vi "SDI_Single-Axis_Test.vi"() -> ()   [LabVIEW 2014]
uses:
  <vilib>/Motion/plugins/PluginFramework/nismSDIFramework.SetFrameworkMode.single.vi
  <vilib>/Motion/Express/_s/nimc.ex.clearFaults.clearFaults.axis.vi
  <vilib>/Motion/Express/_s/nimc.ex.power.power.axis.vi
  <vilib>/Motion/BlockNode/FB.NIMotion.xnode
  <vilib>/Motion/plugins/Delta ASDA SDI Plug-in/Template SoftMotion Drive Interface Plug-in Class.lvclass
panel:
  out "error out":errorcluster
  in  "stop":bool
  in  "Axis":refnum<k21>="Axis 1"
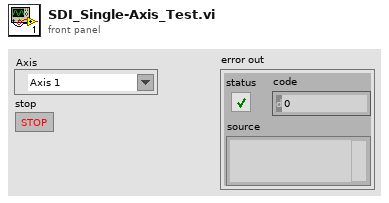
[diagram p1: front panel]
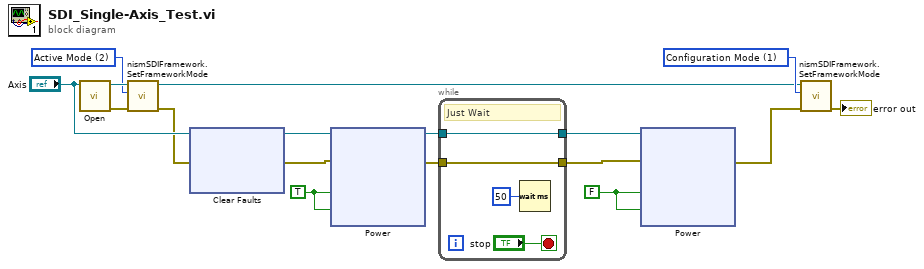
[diagram p0: block diagram]
diagram:
  w8 = 1 items=["Configuration Mode"=1, "Active Mode"=2] ("mode (Active Mode)")
  w11 = FALSE ("enable axis")
  w14 = TRUE ("enable axis")
  w16 = 2 items=["Configuration Mode"=1, "Active Mode"=2] ("mode (Active Mode)")
  n1 = call <vilib>:"Open.vi"("Axis"="Axis") -> ("error out"=w15:errorcluster, "Base Axis Out"=w17:refnum<class "nismPluginAxisBaseClass.lvclass">)  [unwired: 9 in]
  n2 = call-poly <vilib>:"nismSDIFramework.SetFrameworkMode.vi"("error in (no error)"=w15, "mode (Active Mode)"=w16, "Base Axis In"=w17) -> ("error out"=w3:errorcluster, "Base Axis Out"=w7:refnum<class "nismPluginAxisBaseClass.lvclass">)  [unwired: 7 in]
  n3 = xnode ("Clear Faults")("resource"="Axis", "error in"=w3) -> ("resource out"=w2:refnum<k21>, "error out"=w1:errorcluster)
  n4 = xnode ("Power")("enable axis"=w14, "enable drive"=w14, "resource"=w2, "error in"=w1) -> ("resource out"=w12:refnum<k21>, "error out"=w13:errorcluster)
  n5 = while {
    tunnel: w13 -> [w18]
    tunnel: w12 -> [w19]
    tunnel: [w19] -> w10
    tunnel: [w18] -> w9
    stop <- "stop" stop-if-true
    # "Just Wait"
    n6 = Wait (ms)(milliseconds to wait=u32 50) -> ()  [unwired: 1 out]
  }
  n7 = xnode ("Power")("enable axis"=w11, "enable drive"=w11, "resource"=w10, "error in"=w9) -> ("error out"=w6:errorcluster)  [unwired: 1 out]
  n8 = call-poly <vilib>:"nismSDIFramework.SetFrameworkMode.vi"("error in (no error)"=w6, "mode (Active Mode)"=w8, "Base Axis In"=w7) -> ("error out"=→"error out":errorcluster)  [unwired: 7 in, 1 out]
